vi "Zadanie 2 Kamil Orze .vi"() -> ()   [LabVIEW 2024]
panel:
  out "STAN":string
  out "MIN":dbl
  out "MAX":dbl
  in  "Zapis":bool
  out "Alarm dó³":bool
  out "Alarm góra":bool
  in  "Próg górny":dbl
  in  "Próg dolny":dbl
  out "T chwilowa":dbl
  out "T Uœredniona":dbl
  out "Temperatura":T1(graph)
  in  "stop":bool
  in  "URL":string
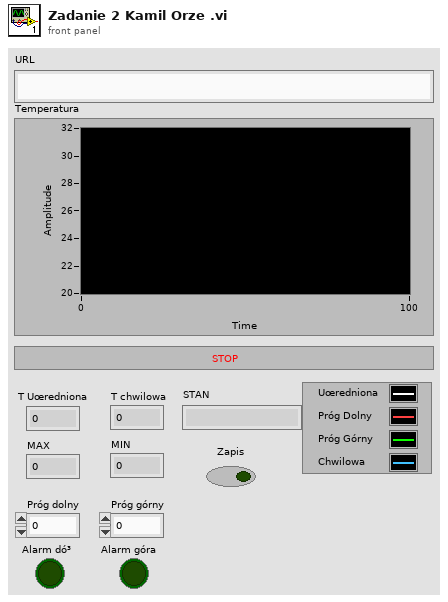
[diagram p1: front panel]
types:
  T1 = cluster{dbl, "Próg dolny":dbl, "próg górny":dbl, dbl}
  T2 = enum16{"Read", "Write", "ReadWrite", "BufferedRead", "BufferedReadWrite"}
  T3 = enum16{"open", "replace", "create", "open or create", "replace or create", "replace or create with confirmation"}
  T4 = cluster{dbl, "Próg dolny":dbl, "Próg górny":dbl, dbl}
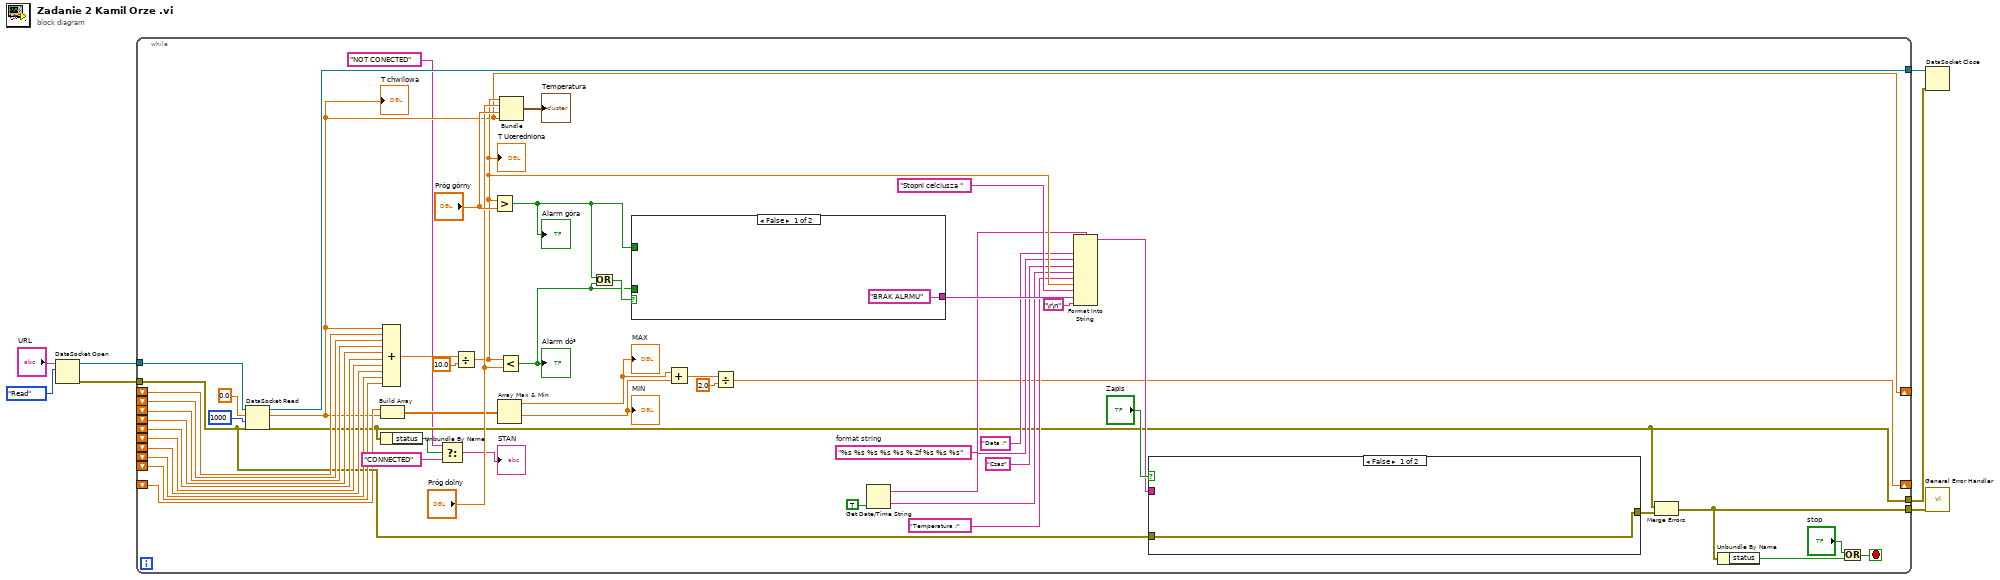
[diagram p0: block diagram]
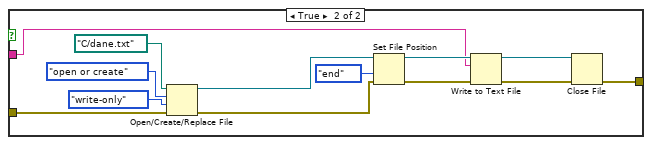
[diagram p2: hidden frame]
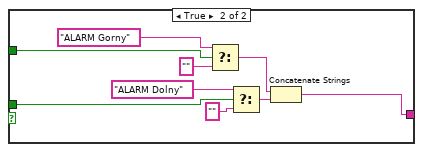
[diagram p3: hidden frame]
diagram:
  n1 = DataSocket Open(10:T2."Read" ("mode"), 11:"URL") -> (0:w4:errorcluster, 3:w6:refnum<k13>)  [unwired: 2 in]
  n2 = while {
    tunnel: w6 -> [w23]
    tunnel: [w22] -> w5
    shift-right: [w10] -> _
    shift-left: _ -> [w58]
    shift-left: _ -> [w57]
    shift-left: _ -> [w56]
    shift-left: _ -> [w55]
    shift-left: _ -> [w54]
    shift-left: _ -> [w53]
    shift-left: _ -> [w52]
    shift-left: _ -> [w51]
    shift-left: _ -> [w50]
    tunnel: w4 -> [w27]
    tunnel: [w14] -> w3
    tunnel: [w24] -> w2
    shift-right: [w11] -> _
    shift-left: _ -> [w20]
    stop <- w35 stop-if-true
    w30 = "%s %s %s %s %s %.2f %s %s %s"  # format string
    n3 = DataSocket Read(8:w27, 9:1000, 10:0.0, 11:w23) -> (0:w14:errorcluster, 2:w10:dbl, 3:w22:refnum<k13>)  [unwired: 1 in, 4 out]
    "T chwilowa" <- w10
    n4 = Build Array "Build Array"(w20, w10) -> (w19:dbl[])
    n5 = Unbundle By Name(w14) -> ("status"=w13:bool)
    n6 = Compound Arithmetic op=ADD(w10, w58, w57, w56, w55, w54, w53, w52, w51, w50) -> (w49:dbl)
    n7 = Select(t="NOT CONECTED", s=w13, f="CONNECTED") -> (s? t:f=→"STAN":string)
    n8 = Divide(x=w49, y=10.0) -> (x/y=w39:dbl)
    "T Uœredniona" <- w39
    n9 = Greater?(x=w39, y="Próg górny") -> (0:w43:bool)
    "Alarm góra" <- w43
    n10 = Array Max & Min(array=w19) -> (max value=w16:dbl, min value=w15:dbl)  [unwired: 2 out]
    "MAX" <- w16
    "MIN" <- w15
    n11 = Less?(x=w39, y="Próg dolny") -> (x < y?=w42:bool)
    "Alarm dó³" <- w42
    n12 = Bundle "Bundle"(w39, "Próg dolny"="Próg dolny", "Próg górny"="Próg górny", w10) -> (→"Temperatura":T4)  [unwired: 1 in]
    n13 = Or(x=w43, y=w42) -> (x .or. y?=w44:bool)
    n14 = case shown="False" w44 {
      tunnel: w43 -> [_ w84]
      tunnel: w42 -> [_ w80]
      tunnel: ["BRAK ALRMU" w78] -> w41
      frame False {
      }
      frame True {
        n15 = Select(t="ALARM Gorny", s=w84, f="") -> (s? t:f=w76:string)
        n16 = Select(t="ALARM Dolny", s=w80, f="") -> (s? t:f=w77:string)
        n17 = Concatenate Strings "Concatenate Strings"(w76, w77) -> (w78:string)
      }
    }
    n18 = Add(x=w16, y=w15) -> (x+y=w18:dbl)
    n19 = Divide(x=w18, y=2.0) -> (x/y=w11:dbl)
    n20 = Get Date/Time String(want seconds? (F)=TRUE) -> (date string=w33:string, time string=w31:string)  [unwired: 2 in]
    n21 = Format Into String(format string=w30, "Data :", w33, "Czas", w31, "Temperatura :", w39, "Stopni celciusza ", w41, "\r\n") -> (resulting string=w21:string)  [unwired: 2 in, 1 out]
    n22 = case shown="False" "Zapis" {
      tunnel: w27 -> [w61 w71]
      tunnel: [w61 w63] -> w28
      tunnel: w21 -> [_ w62]
      frame False {
      }
      frame True {
        n23 = Open/Create/Replace File(file path (use dialog)=path "C:/dane.txt", error in=w71, operation (0:open)=T3."open or create", access (0:read/write)=enum16{"read/write", "read-only", "write-only"}."write-only") -> (refnum out=w69:refnum<file>, error out=w70:errorcluster)  [unwired: 2 in, 1 out]
        n24 = Set File Position(refnum=w69, from (0:start)=enum16{"start", "end", "current"}."end", error in=w70) -> (refnum out=w65:refnum<file>, error out=w67:errorcluster)  [unwired: 1 in]
        n25 = Write to Text File(file (use dialog)=w65, text=w62, error in=w67) -> (refnum out=w64:refnum<file>, error out=w66:errorcluster)  [unwired: 1 in, 1 out]
        n26 = Close File(refnum=w64, error in=w66) -> (error out=w63:errorcluster)  [unwired: 1 out]
      }
    }
    n27 = Merge Errors "Merge Errors"(w14, w28) -> (w24:errorcluster)
    n28 = Unbundle By Name "Unbundle By Name"(w24) -> ("status"=w25:bool)
    n29 = Or(x="stop", y=w25) -> (x .or. y?=w35:bool)
  }
  n30 = DataSocket Close(8:w3, 11:w5) -> ()  [unwired: 1 in, 2 out]
  n31 = call <vilib>:"General Error Handler.vi"("error in (no error)"=w2) -> ()  [unwired: 10 in, 5 out]
